vi "Convert Encoder to Angle v2.vi"(11 "Encoder Units":dbl) -> (0 "Floor":dbl, 3 "Angle":dbl)   [LabVIEW 2017]
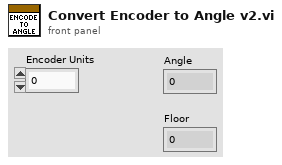
[diagram p1: front panel]
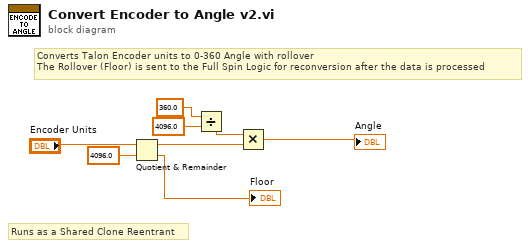
[diagram p0: block diagram]
diagram:
  # "Runs as a Shared Clone Reentrant"
  # "Converts Talon Encoder units to 0-360 Angle with rollover\nThe Rollover (Floor) is sent to the Full Spin Logic for reconversion after the data is processed"
  n1 = Quotient & Remainder(x="Encoder Units", y=4096.0) -> (x-y*floor(x/y)=w5:dbl, floor(x/y)=→"Floor":dbl)
  n2 = Divide(x=360.0, y=4096.0) -> (x/y=w4:dbl)
  n3 = Multiply(x=w4, y=w5) -> (x*y=→"Angle":dbl)
